vi "Basic Hunt Mode.vi"(2 "Us Y":dbl, 3 "Us X":dbl, 4 "Nav String":string="$,G,43,13,230,P,10,20,120,T,10,10,330,L,14,36,110,A,3,5,B,7,8,C,16,20,D,-1,-1,S,08,12,234\r", 5 "Target":string="P") -> (0 "YGoal":i32, 1 "XGoal":i32)   [LabVIEW 2012]
panel:
  out "Tug Y":i32
  out "Tug X":i32
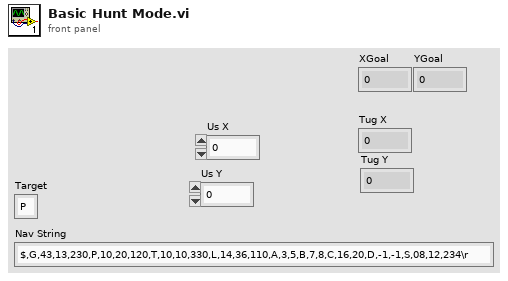
[diagram p1: front panel]
types:
  T1 = cluster{"regular expression":string, i32, i32, i32}
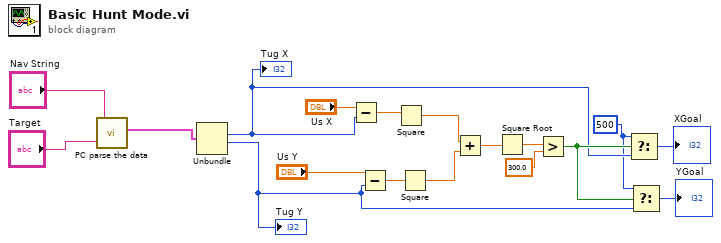
[diagram p0: block diagram]
diagram:
  w3 = 500 ("t")
  n1 = call "PC parse the data.vi"("Nav String"="Nav String", "Tug"="Target") -> ("Tug Location"=w17:T1)  [unwired: 3 out]
  n2 = Unbundle(w17) -> (w4:i32, w5:i32)  [unwired: 2 out]
  "Tug X" <- w4
  "Tug Y" <- w5
  n3 = Subtract(x="Us X", y=w4) -> (x-y=w12:dbl)
  n4 = Subtract(x="Us Y", y=w5) -> (x-y=w13:dbl)
  n5 = Square(x=w12) -> (x^2=w10:dbl)
  n6 = Square(x=w13) -> (x^2=w11:dbl)
  n7 = Add(x=w10, y=w11) -> (x+y=w9:dbl)
  n8 = Square Root(x=w9) -> (sqrt(x)=w8:dbl)
  n9 = Greater?(x=w8, y=300.0) -> (0:w6:bool)
  n10 = Select(t=w3, s=w6, f=w4) -> (s? t:f=→"XGoal":i32)
  n11 = Select(t=w3, s=w6, f=w5) -> (s? t:f=→"YGoal":i32)
